vi "Login in.vi"(8 "error in (no error)":errorcluster) -> (0 "error out":errorcluster, 3 "Pass?":bool)   [LabVIEW 2017, in "Toolbox.lvlib"]
uses:
  Toolbox.lvlib
panel:
  in  "Cancel Button":bool
  in  "OK Button":bool
  in  "Password":string
  # "Password:"
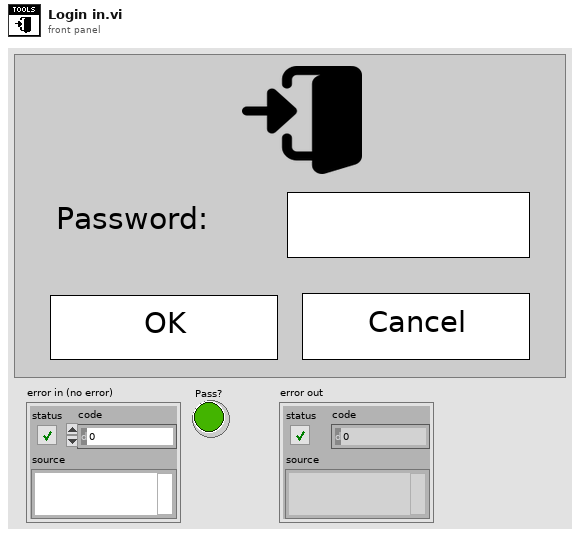
[diagram p1: front panel]
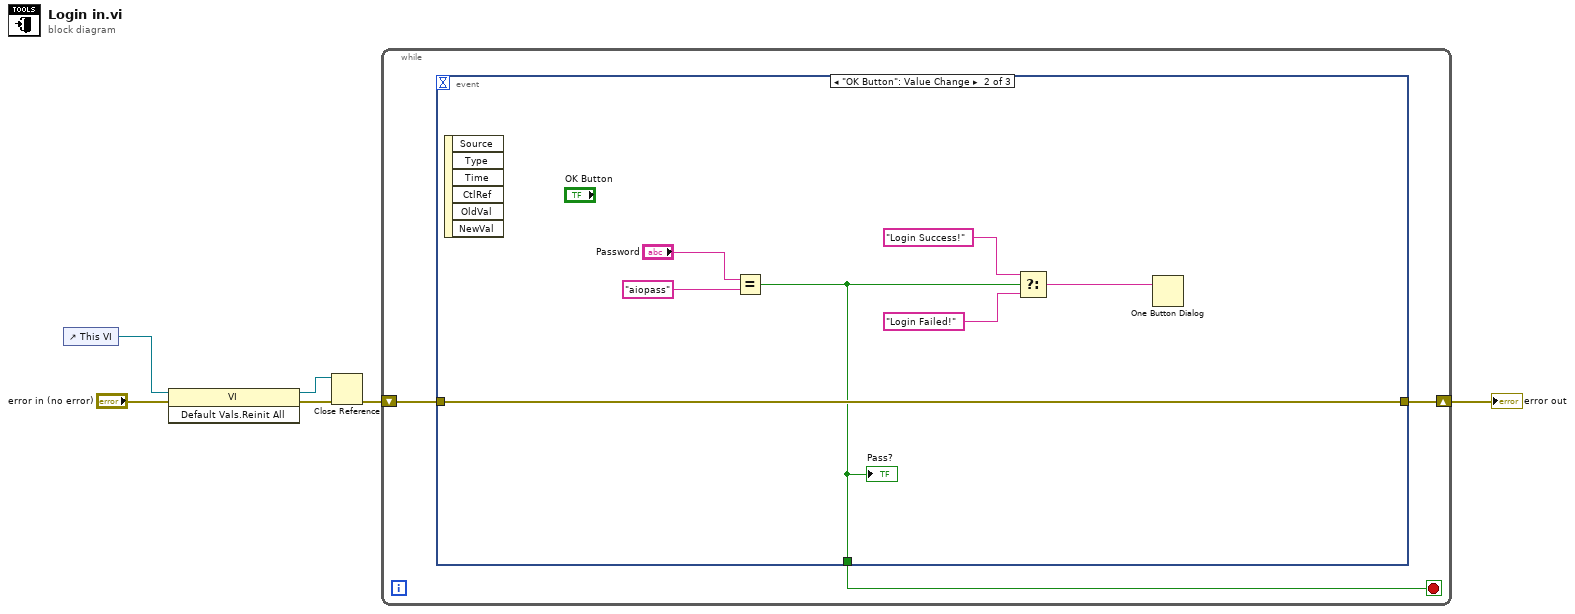
[diagram p0: block diagram]
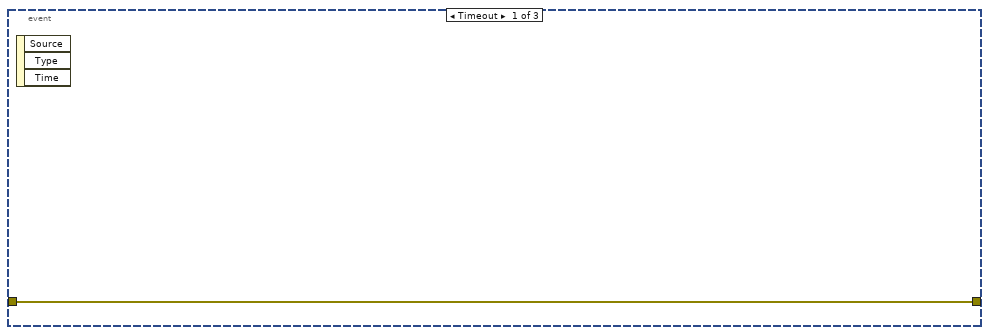
[diagram p2: hidden frame]
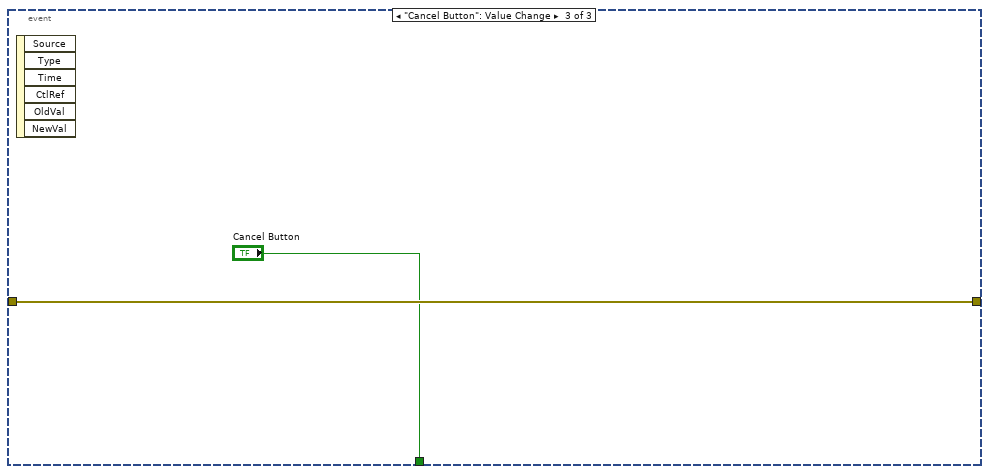
[diagram p3: hidden frame]
diagram:
  n1 = control-ref of="This VI"() -> (w3:refnum<vi>)
  n2 = invoke class="VI" method="Default Vals.Reinit All"(reference=w3, error in="error in (no error)") -> (reference out=w1:refnum<vi>, error out=w4:errorcluster)  [unwired: 1 in, 1 out]
  n3 = Close Reference(reference=w1, error in (no error)=w4) -> (error out=w2:errorcluster)
  n4 = while {
    shift-right: [w8] -> w5
    shift-left: w2 -> [w9]
    stop <- w7 stop-if-true
    n5 = event shown="[1] \"OK Button\": Value Change" {
      selector: _ -> [_ _ _]
      dyn-events: _ -> [_ _ _]
      timeout: _ -> [_ _ _]
      tunnel: w9 -> [w10 w15 w19]
      tunnel: [w10 w15 w19] -> w8
      tunnel: [_ w11 "Cancel Button"] -> w7
      event Timeout {
        n6 = event-data() -> ()  [unwired: 1 in, 3 out]
      }
      event "OK Button": Value Change {
        n7 = event-data() -> ()  [unwired: 1 in, 6 out]
        n8 = Equal?(x="Password", y="aiopass") -> (x = y?=w11:bool)
        "Pass?" <- w11
        n9 = Select(t="Login Success!", s=w11, f="Login Failed!") -> (s? t:f=w12:string)
        n10 = One Button Dialog(message=w12) -> ()  [unwired: 1 in, 1 out]
      }
      event "Cancel Button": Value Change {
        n11 = event-data() -> ()  [unwired: 1 in, 6 out]
      }
    }
  }
  "error out" <- w5
